vi "Check.vi"(8 "error in (no error)":errorcluster, 11 "Pound":refnum<class "Pound.lvclass">) -> (0 "error out":errorcluster, 1 "Watchdog Name":string, 2 "ExpirationType":T1, 3 "Pound":refnum<class "Pound.lvclass">)   [LabVIEW 2017, in "Pound.lvclass"]
doc: "Checks if any of the watchdogs have expired."
uses:
  <vilib>/NI/Software Watchdog/Pound/Pound.lvclass
  <vilib>/NI/Software Watchdog/Pound/ExpirationType.ctl
  <vilib>/NI/Software Watchdog/Pound/Pound.lvclass/Pound.ctl
  <vilib>/NI/Software Watchdog/Watchdog/Watchdog.lvclass
  <vilib>/NI/Software Watchdog/Watchdog/Read Shutdown Timeout.vi
  <vilib>/NI/Software Watchdog/Watchdog/Read Name.vi
  <vilib>/NI/Software Watchdog/Pound/Read Shutdown Timestamp.vi
  <vilib>/NI/Software Watchdog/Pound/Read Mode.vi
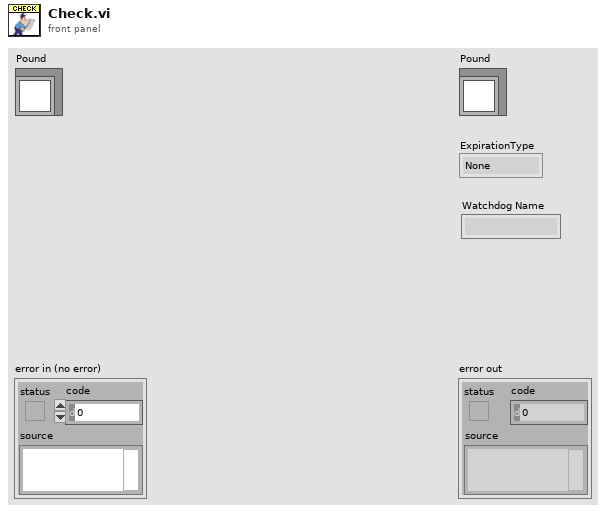
[diagram p1: front panel]
types:
  T1 = typedef "Pound.lvclass/ExpirationType.ctl" = enum16{"None", "Execution", "Shutdown"}
  T2 = typedef "Pound.lvclass/Status.ctl" = cluster{"WatchdogName":string, "ExpirationType":T1}
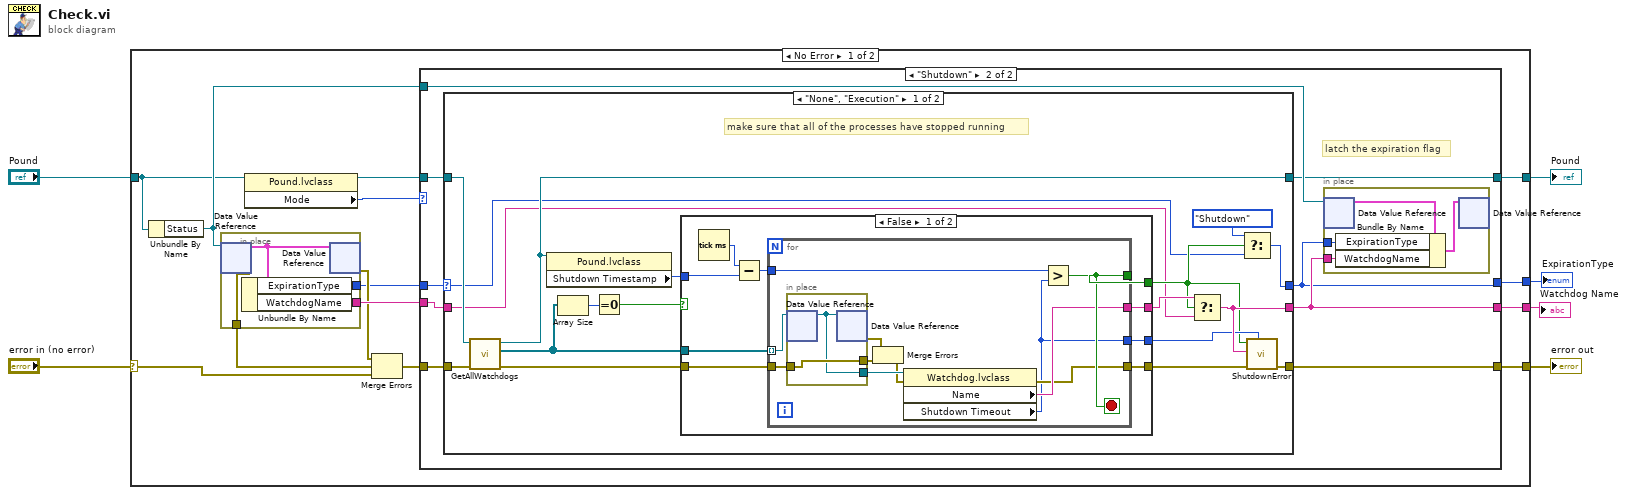
[diagram p0: block diagram]
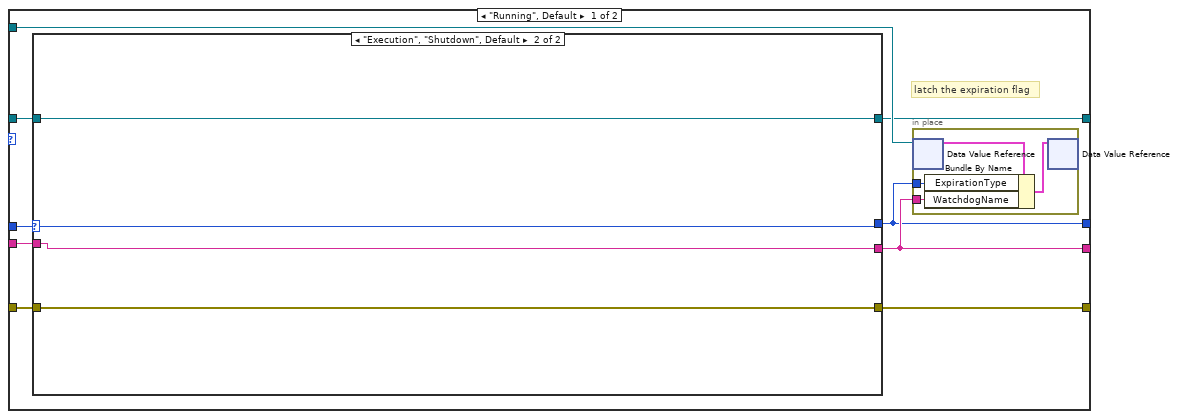
[diagram p2: hidden frame]
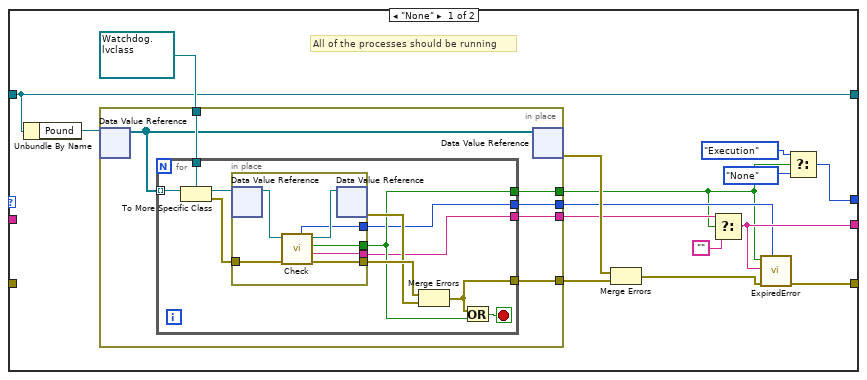
[diagram p3: hidden frame]
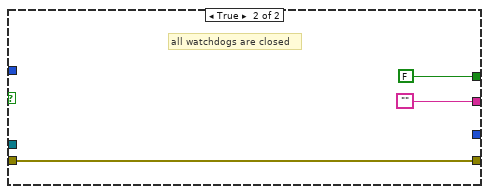
[diagram p4: hidden frame]
diagram:
  n1 = case shown="No Error" "error in (no error)" {
    selector: "error in (no error)" -> [w7 w142]
    tunnel: [w20 w142] -> w5
    tunnel: [w19 w141] -> w3
    tunnel: "Pound" -> [w12 w141]
    tunnel: [w18 _] -> w2
    tunnel: [w8 _] -> w1
    frame No Error {
      n2 = Unbundle By Name(w12) -> ("Status"=w16:refnum<data-value>)
      n3 = in-place {
        in-place-border: [w24] -> w9
        in-place-border: [w23] -> w17
        in-place-border: [w21] -> w13
        n4 = in-place-dvr #1(w16) -> (w22:T2, w21:errorcluster)
        n5 = Unbundle By Name(w22) -> ("ExpirationType"=w24:T1, "WatchdogName"=w23:string)
        n6 = in-place-dvr #1(w22) -> (w15:errorcluster)  [unwired: 1 out]
      }
      n7 = property class="Pound.lvclass"(reference=w12) -> (reference out=w11:refnum<class "Pound.lvclass">, "Mode"=w10:enum16{"Running", "Shutdown"})  [unwired: 1 in, 1 out]
      n8 = Merge Errors(w15, w13, w7) -> (w14:errorcluster)
      n9 = case shown="\"Shutdown\"" w10 {
        tunnel: [w28 w84] -> w20
        tunnel: w11 -> [w31 w87]
        tunnel: [w29 w85] -> w19
        tunnel: [w32 w88] -> w18
        tunnel: w17 -> [w25 w82]
        tunnel: w14 -> [w30 w86]
        tunnel: w16 -> [w33 w89]
        tunnel: w9 -> [w27 w83]
        tunnel: [w26 w81] -> w8
        frame "Running", Default {
          # "latch the expiration flag"
          n10 = case shown="\"Execution\", \"Shutdown\", Default" w27 {
            selector: w27 -> [_ w75]
            tunnel: [w44 w73] -> w28
            tunnel: [w34 w75] -> w26
            tunnel: [w42 w74] -> w32
            tunnel: w31 -> [w40 w76]
            tunnel: w30 -> [_ w73]
            tunnel: [w40 w76] -> w29
            tunnel: w25 -> [_ w74]
            frame "None" {
              # "All of the processes should be running"
              n11 = Unbundle By Name(w40) -> ("Pound"=w39:refnum<data-value>)
              n12 = in-place {
                in-place-border: [w54] -> w47
                in-place-border: [w53] -> w37
                in-place-border: [w52] -> w43
                in-place-border: refnum<data-value> refnum ("data value reference") -> [w51]
                in-place-border: [w49] -> w38
                n13 = in-place-dvr #2(w39) -> (w50:refnum<data-value>[])  [unwired: 1 out]
                n14 = for {
                  tunnel: w50 -> [w65] mode=indexing
                  tunnel: [w59] -> w54
                  tunnel: [w58] -> w53
                  tunnel: [w57] -> w52
                  tunnel: w51 -> [w56]
                  tunnel: [w55] -> w49
                  stop <- w63 stop-if-true
                  n15 = To More Specific Class(target class=w56, reference=w65) -> (specific class reference=w64:refnum<data-value>, error out=w62:errorcluster)  [unwired: 1 in]
                  n16 = in-place {
                    in-place-border: [w71] -> w58
                    in-place-border: [w70] -> w57
                    in-place-border: [w69] -> w61
                    in-place-border: w62 -> [w67]
                    in-place-border: [w66] -> w55
                    n17 = in-place-dvr #3(w64) -> (w72:refnum<class "Watchdog.lvclass">)  [unwired: 1 out]
                    n18 = call <vilib>:"Check.vi"("error in (no error)"=w67, "Watchdog in"=w72) -> ("error out"=w69:errorcluster, "Watchdog Name"=w70:string, "Expired"=w71:bool, "Watchdog out"=w68:refnum<class "Watchdog.lvclass">, "Execution Timeout"=w66:u32)  [unwired: 5 in]
                    n19 = in-place-dvr #3(w68) -> (w60:errorcluster)  [unwired: 1 out]
                  }
                  n20 = Merge Errors(w61, w60) -> (w59:errorcluster)
                  n21 = Or(x=w59, y=w58) -> (x .or. y?=w63:bool)
                }
                n22 = in-place-dvr #2(w50) -> (w46:errorcluster)  [unwired: 1 out]
              }
              n23 = Merge Errors(w46, w47) -> (w45:errorcluster)
              n24 = Select(t=w43, s=w37, f="") -> (s? t:f=w42:string)
              n25 = call <vilib>:"ExpiredError.vi"("Timeout"=w38, "error in (no error)"=w45, "Watchdog Name"=w42, "Expired"=w37) -> ("error out"=w44:errorcluster)  [unwired: 7 in]
              n26 = Select(t=ExpirationType."Execution" ("ExpirationType"), s=w37, f=ExpirationType."None" ("ExpirationType")) -> (s? t:f=w34:T1)
            }
            frame "Execution", "Shutdown", Default {
            }
          }
          n27 = in-place {
            in-place-border: w32 -> [w78]
            in-place-border: w26 -> [w77]
            n28 = in-place-dvr #4(w33) -> (w80:T2)  [unwired: 1 out]
            n29 = Bundle By Name(cluster=w80, "ExpirationType"=w77, "WatchdogName"=w78) -> (w79:T2)
            n30 = in-place-dvr #4(w79) -> ()  [unwired: 2 out]
          }
        }
        frame "Shutdown" {
          # "latch the expiration flag"
          n31 = case shown="\"None\", \"Execution\"" w83 {
            selector: w83 -> [w91 w135]
            tunnel: [w98 w133] -> w84
            tunnel: [w96 w134] -> w88
            tunnel: w87 -> [w107 w136]
            tunnel: w86 -> [w106 w133]
            tunnel: [w101 w136] -> w85
            tunnel: [w93 w135] -> w81
            tunnel: w82 -> [w90 w134]
            frame "None", "Execution" {
              # "make sure that all of the processes have stopped running"
              n32 = call <vilib>:"GetAllWatchdogs.vi"("error in (no error)"=w106, "Pound in"=w107) -> ("error out"=w102:errorcluster, "All Watchdogs"=w103:refnum<data-value>[], "Pound out"=w101:refnum<class "Pound.lvclass">)  [unwired: 7 in]
              n33 = property class="Pound.lvclass"(reference=w101) -> ("Shutdown Timestamp"=w100:u32)  [unwired: 1 in, 2 out]
              n34 = Array Size(array=w103) -> (size(s)=w105:i32)
              n35 = Equal To 0?(x=w105) -> (x = 0?=w104:bool)
              n36 = case shown="False" w104 {
                tunnel: w103 -> [w115 _]
                tunnel: w102 -> [w116 w130]
                tunnel: w100 -> [w113 _]
                tunnel: [w111 FALSE] -> w94
                tunnel: [w110 ""] -> w97
                tunnel: [w109 w130] -> w99
                tunnel: [w108 _] -> w95
                frame False {
                  n37 = Tick Count (ms)() -> (millisecond timer value=w114:u32)
                  n38 = Subtract(x=w114, y=w113) -> (x-y=w112:u32)
                  n39 = for {
                    tunnel: w116 -> [w126]
                    tunnel: w115 -> [w127] mode=indexing
                    tunnel: w112 -> [w125]
                    tunnel: [w124] -> w111
                    tunnel: [w120] -> w110
                    tunnel: [w118] -> w109
                    tunnel: [w117] -> w108
                    stop <- w124 stop-if-true
                    n40 = in-place {
                      in-place-border: w126 -> [w129]
                      in-place-border: [w128] -> w121
                      in-place-border: [w129] -> w122
                      n41 = in-place-dvr #5(w127) -> (w128:refnum<class "Watchdog.lvclass">)  [unwired: 1 out]
                      n42 = in-place-dvr #5(w128) -> (w123:errorcluster)  [unwired: 1 out]
                    }
                    n43 = Merge Errors(w123, w122) -> (w119:errorcluster)
                    n44 = property class="Watchdog.lvclass"(reference=w121, error in=w119) -> (error out=w118:errorcluster, "Name"=w120:string, "Shutdown Timeout"=w117:u32)  [unwired: 1 out]
                    n45 = Greater?(x=w125, y=w117) -> (0:w124:bool)
                  }
                }
                frame True {
                  # "all watchdogs are closed"
                }
              }
              n46 = Select(t=w97, s=w94, f=w90) -> (s? t:f=w96:string)
              n47 = Select(t=ExpirationType."Shutdown" ("ExpirationType"), s=w94, f=w91) -> (s? t:f=w93:T1)
              n48 = call <vilib>:"ShutdownError.vi"("Timeout"=w95, "error in (no error)"=w99, "Watchdog Name"=w96, "Expired"=w94) -> ("error out"=w98:errorcluster)  [unwired: 7 in]
            }
            frame "Shutdown", Default {
            }
          }
          n49 = in-place {
            in-place-border: w88 -> [w138]
            in-place-border: w81 -> [w137]
            n50 = in-place-dvr #6(w89) -> (w140:T2)  [unwired: 1 out]
            n51 = Bundle By Name(cluster=w140, "ExpirationType"=w137, "WatchdogName"=w138) -> (w139:T2)
            n52 = in-place-dvr #6(w139) -> ()  [unwired: 2 out]
          }
        }
      }
    }
    frame Error {
    }
  }
  "error out" <- w5
  "Pound" <- w3
  "Watchdog Name" <- w2
  "ExpirationType" <- w1
